vi "Fetch Measurement - WaveformMode.vi"(8 "error in":errorcluster, 11 "Waveform Mode - Control":T1) -> (0 "error out":errorcluster, 3 "Waveform Mode - Result":T1)   [LabVIEW 2021, in "Waveform Mode_Channel Ganging.lvlib"]
uses:
  Waveform Mode_Channel Ganging.lvlib
  Controls/Waveform Mode Measurement.ctl
  shared subVIs/ctl/NIDCPower_channel_ganging - ctl - ganged session.ctl
  shared subVIs/ctl/NIDCPower_channel_ganging - ctl - ganged config.ctl
  shared subVIs/ctl/NIDCPower_channel_ganging - ctl - channel mode.ctl
  Measurement Results.ctl
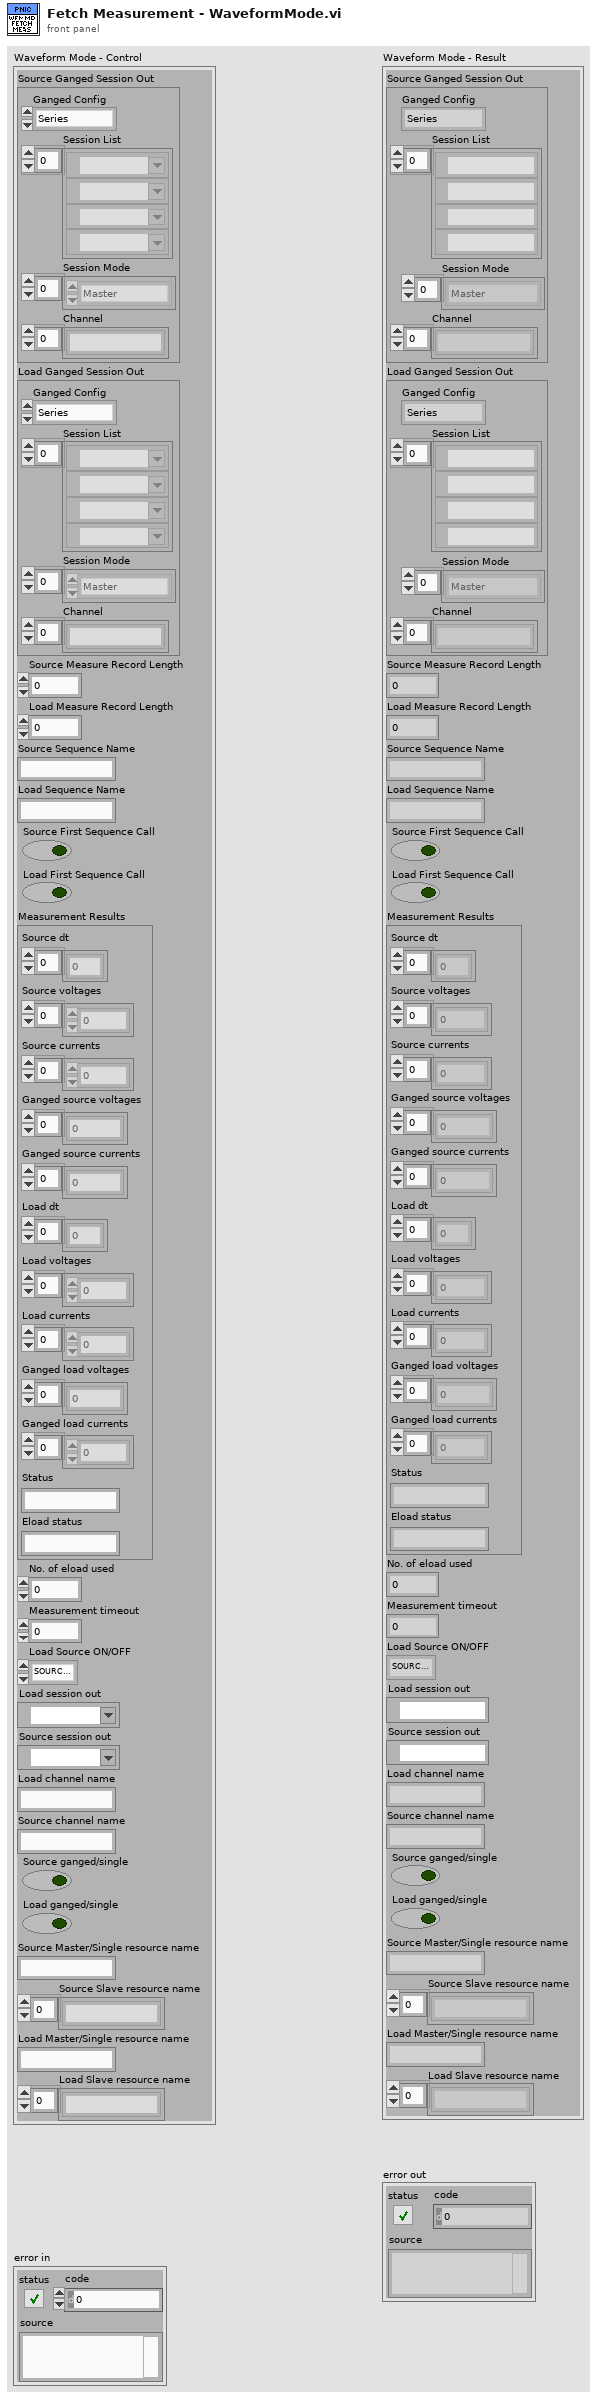
[diagram p1: front panel]
types:
  T1 = typedef "Waveform Mode_Channel Ganging.lvlib/Waveform Mode Measurement.ctl" = cluster{"Source Ganged Session Out":T2, "Load Ganged Session Out":T2, "Source Measure Record Length":i32, "Load Measure Record Length":i32, "Source Sequence Name":string, "Load Sequence Name":string, "Source First Sequence Call":bool, "Load First Sequence Call":bool, "Measurement Results":T5, "No. of eload used":i32, "Measurement timeout":dbl, "Load Source ON/OFF":enum16{"SOURCE AND LOAD OFF", "SOURCE ON", "LOAD ON", "SOURCE AND LOAD ON"}, "Load session out":refnum<k15>, "Source session out":refnum<k15>, "Load channel name":string, "Source channel name":string, "Source ganged/single":bool, "Load ganged/single":bool, "Source Master/Single resource name":string, "Source Slave resource name":string[], "Load Master/Single resource name":string, "Load Slave resource name":string[]}
  T2 = typedef "NIDCPower_channel_ganging - ctl - ganged session.ctl" = cluster{"Ganged Config":T3, "Session List":refnum<k15>[], "Session Mode":T4[], "Channel":string[]}
  T3 = typedef "NIDCPower_channel_ganging - ctl - ganged config.ctl" = enum32{"Series", "Parallel", "Manual"}
  T4 = typedef "NIDCPower_channel_ganging - ctl - channel mode.ctl" = enum32{"Master", "Slave", "Slave - Inverted"}
  T5 = typedef "Waveform Mode_Channel Ganging.lvlib/Measurement Results.ctl" = cluster{"Source dt":dbl[], "Source voltages":dbl[], "Source currents":dbl[], "Ganged source voltages":dbl[], "Ganged source currents":dbl[], "Load dt":dbl[], "Load voltages":dbl[], "Load currents":dbl[], "Ganged load voltages":dbl[], "Ganged load currents":dbl[], "Status":string, "Eload status":string}
  T6 = enum16{"SOURCE AND LOAD OFF", "SOURCE ON", "LOAD ON", "SOURCE AND LOAD ON"}
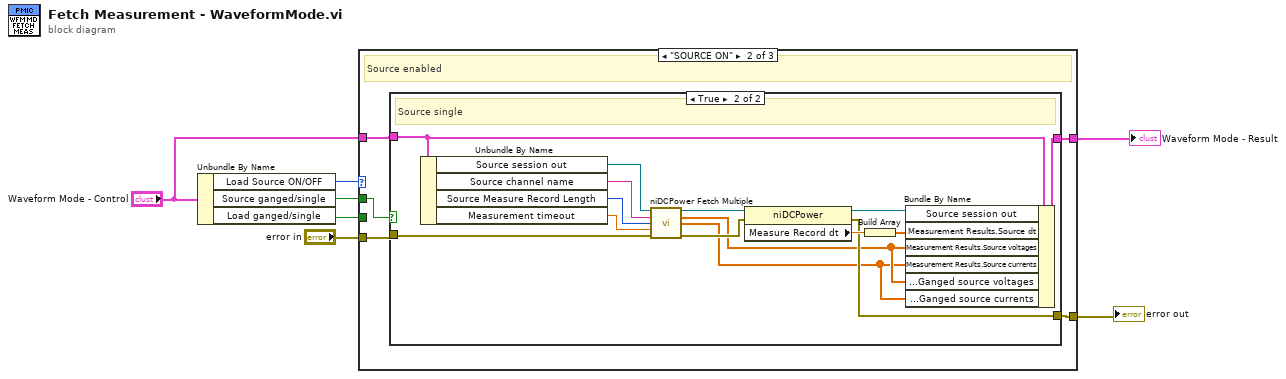
[diagram p0: block diagram]
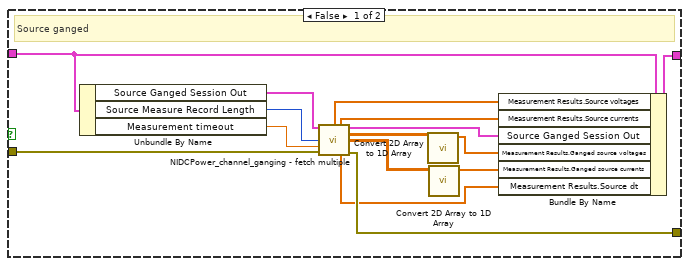
[diagram p3: hidden frame]
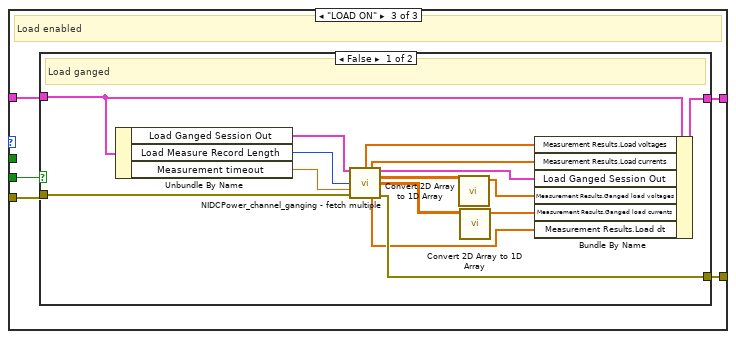
[diagram p4: hidden frame]
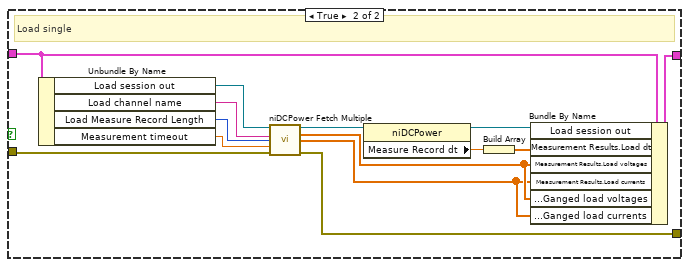
[diagram p5: hidden frame]
diagram:
  n1 = Unbundle By Name("Waveform Mode - Control") -> ("Load Source ON/OFF"=w2:T6, "Source ganged/single"=w3:bool, "Load ganged/single"=w4:bool)
  n2 = case shown="\"SOURCE ON\"" w2 {
    tunnel: "Waveform Mode - Control" -> [w9 w11 w47]
    tunnel: [w9 w14 w46] -> w6
    tunnel: [w8 w13 w45] -> w7
    tunnel: "error in" -> [w8 w12 w49]
    tunnel: w3 -> [_ w10 _]
    tunnel: w4 -> [_ _ w48]
    frame Default {
    }
    frame "SOURCE ON" {
      # "Source enabled"
      n3 = case shown="True" w10 {
        tunnel: w12 -> [w25 w42]
        tunnel: w11 -> [w15 w41]
        tunnel: [w29 w40] -> w14
        tunnel: [w24 w32] -> w13
        frame False {
          # "Source ganged"
          n4 = Unbundle By Name(w15) -> ("Source Ganged Session Out"=w28:T2, "Source Measure Record Length"=w26:i32, "Measurement timeout"=w27:dbl)
          n5 = call "NIDCPower_channel_ganging - fetch multiple.vi"("Ganged Session In"=w28, "Count"=w26, "timeout (1.0)"=w27, "error in (no error)"=w25) -> ("Ganged Voltage Measurement"=w17:dbl[], "Ganged Current Measurement"=w16:dbl[], "Ganged Session Out"=w22:T2, "voltage measurements"=w21:dbl[][], "current measurements"=w20:dbl[][], "Measure Record dt"=w23:dbl[], "error out"=w24:errorcluster)  [unwired: 4 in, 1 out]
          n6 = call "Convert 2D Array to 1D Array.vi"("Array in"=w21) -> ("Array out"=w19:dbl[])  [unwired: 10 in]
          n7 = call "Convert 2D Array to 1D Array.vi"("Array in"=w20) -> ("Array out"=w18:dbl[])  [unwired: 10 in]
          n8 = Bundle By Name(cluster=w15, "Measurement Results.Source voltages"=w17, "Measurement Results.Source currents"=w16, "Source Ganged Session Out"=w22, "Measurement Results.Ganged source voltages"=w19, "Measurement Results.Ganged source currents"=w18, "Measurement Results.Source dt"=w23) -> (w29:T1)
        }
        frame True {
          # "Source single"
          n9 = Unbundle By Name(w41) -> ("Source session out"=w44:refnum<k15>, "Source channel name"=w43:string, "Source Measure Record Length"=w34:i32, "Measurement timeout"=w39:dbl)
          n10 = call <instrlib>:"niDCPower Fetch Multiple.vi"("instrument handle"=w44, "channel name"=w43, "count (1)"=w34, "timeout (1.0)"=w39, "error in (no error)"=w42) -> ("instrument handle out"=w38:refnum<k15>, "voltage measurements"=w31:dbl[], "current measurements"=w30:dbl[], "error out"=w33:errorcluster)  [unwired: 7 out]
          n11 = property class="niDCPower"(reference=w38, error in=w33) -> (reference out=w37:refnum<k15>, error out=w32:errorcluster, "Measure Record dt"=w36:dbl)
          n12 = Build Array(w36) -> (w35:dbl[])
          n13 = Bundle By Name(cluster=w41, "Source session out"=w37, "Measurement Results.Source dt"=w35, "Measurement Results.Source voltages"=w31, "Measurement Results.Source currents"=w30, "Measurement Results.Ganged source voltages"=w31, "Measurement Results.Ganged source currents"=w30) -> (w40:T1)
        }
      }
    }
    frame "LOAD ON" {
      # "Load enabled"
      n14 = case shown="False" w48 {
        tunnel: w49 -> [w60 w76]
        tunnel: w47 -> [w50 w74]
        tunnel: [w64 w73] -> w46
        tunnel: [w59 w75] -> w45
        frame False {
          # "Load ganged"
          n15 = Unbundle By Name(w50) -> ("Load Ganged Session Out"=w63:T2, "Load Measure Record Length"=w61:i32, "Measurement timeout"=w62:dbl)
          n16 = call "NIDCPower_channel_ganging - fetch multiple.vi"("Ganged Session In"=w63, "Count"=w61, "timeout (1.0)"=w62, "error in (no error)"=w60) -> ("Ganged Voltage Measurement"=w52:dbl[], "Ganged Current Measurement"=w51:dbl[], "Ganged Session Out"=w57:T2, "voltage measurements"=w56:dbl[][], "current measurements"=w55:dbl[][], "Measure Record dt"=w58:dbl[], "error out"=w59:errorcluster)  [unwired: 4 in, 1 out]
          n17 = call "Convert 2D Array to 1D Array.vi"("Array in"=w56) -> ("Array out"=w54:dbl[])  [unwired: 10 in]
          n18 = call "Convert 2D Array to 1D Array.vi"("Array in"=w55) -> ("Array out"=w53:dbl[])  [unwired: 10 in]
          n19 = Bundle By Name(cluster=w50, "Measurement Results.Load voltages"=w52, "Measurement Results.Load currents"=w51, "Load Ganged Session Out"=w57, "Measurement Results.Ganged load voltages"=w54, "Measurement Results.Ganged load currents"=w53, "Measurement Results.Load dt"=w58) -> (w64:T1)
        }
        frame True {
          # "Load single"
          n20 = Unbundle By Name(w74) -> ("Load session out"=w78:refnum<k15>, "Load channel name"=w77:string, "Load Measure Record Length"=w67:i32, "Measurement timeout"=w72:dbl)
          n21 = call <instrlib>:"niDCPower Fetch Multiple.vi"("instrument handle"=w78, "channel name"=w77, "count (1)"=w67, "timeout (1.0)"=w72, "error in (no error)"=w76) -> ("instrument handle out"=w71:refnum<k15>, "voltage measurements"=w66:dbl[], "current measurements"=w65:dbl[], "error out"=w75:errorcluster)  [unwired: 7 out]
          n22 = property class="niDCPower"(reference=w71) -> (reference out=w70:refnum<k15>, "Measure Record dt"=w69:dbl)  [unwired: 1 in, 1 out]
          n23 = Build Array(w69) -> (w68:dbl[])
          n24 = Bundle By Name(cluster=w74, "Load session out"=w70, "Measurement Results.Load dt"=w68, "Measurement Results.Load voltages"=w66, "Measurement Results.Load currents"=w65, "Measurement Results.Ganged load voltages"=w66, "Measurement Results.Ganged load currents"=w65) -> (w73:T1)
        }
      }
    }
  }
  "error out" <- w7
  "Waveform Mode - Result" <- w6
